vi "Transform_Create_TransRot.vi"(9 "ROTATION":T3, 11 "TRANSLATION":T2) -> (3 "TRANSFORM":T1)   [LabVIEW 2019, in "Trajectory_Library.lvlib"]
doc: "Constructs a transform with the given translation and rotation components.\n\nParameters:\n - translation -Translational component of the transform.\n - rotation - Rotational component of the transform.\n\nResult:\n - transform - TRANSFORM data structure"
uses:
  Trajectory_Library.lvlib
  TRANSLATION2D.ctl
  ROTATION2D.ctl
  TRANSFORM2D.ctl
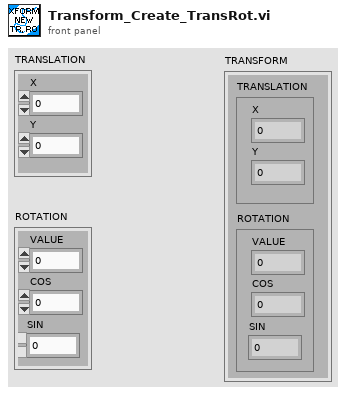
[diagram p1: front panel]
types:
  T1 = typedef "Trajectory_Library.lvlib/TRANSFORM2D.ctl" = cluster{"TRANSLATION":T2, "ROTATION":T3}
  T2 = typedef "Trajectory_Library.lvlib/TRANSLATION2D.ctl" = cluster{"X":dbl, "Y":dbl}
  T3 = typedef "Trajectory_Library.lvlib/ROTATION2D.ctl" = cluster{"VALUE":dbl, "COS":dbl, "SIN":dbl}
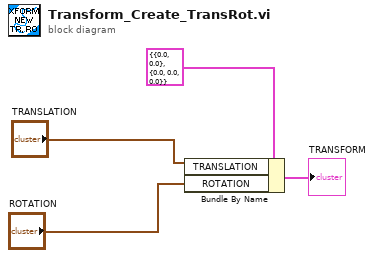
[diagram p0: block diagram]
diagram:
  n1 = Bundle By Name(cluster=T1 {"TRANSLATION"={"X"=0.0, "Y"=0.0}, "ROTATION"={"VALUE"=0.0, "COS"=0.0, "SIN"=0.0}} ("TRANSFORM"), "TRANSLATION"="TRANSLATION", "ROTATION"="ROTATION") -> (→"TRANSFORM":T1)
